vi "RT Main_Write Scalar.vi"() -> ()   [LabVIEW 2018]
uses:
  FPGA Bitfile Register Operations/Scalar IO Operations/TypeDefs/FXP Configuration.ctl
  <vilib>/fxp/LVFixedPointRepBitsTypeDef.ctl
  <vilib>/fxp/LVFixedPointRepRangeTypeDef.ctl
  FPGA Bitfile Register Operations/Scalar IO Operations/Write Methods/Write FXP.vi
  FPGA Bitfile Register Operations/Scalar IO Operations/Read Methods/Read FXP.vi
  <vilib>/FPGAPlugInAG/Dynamic/niLvFpga_Close_Dynamic.vi
  <vilib>/rvi/interface/nirviCloseFPGA/nirviCloseFPGA.xnode
  FPGA Bitfile Register Operations/Scalar IO Operations/Scalar IO Operations.lvlib
panel:
  in  "DBL Value Write":dbl=10.5 format="%#_13g"
  out "DBL Value Out":dbl
  out "Average seconds per write":dbl format="%#_6f"
  out "error out":errorcluster
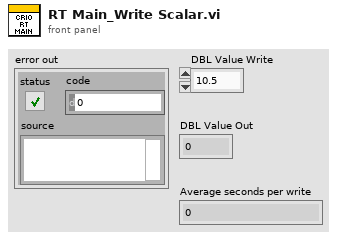
[diagram p1: front panel]
types:
  T1 = typedef "Scalar IO Operations.lvlib/FXP Configuration.ctl" = cluster{"FXP Representation":T2, "FXP Range":T3}
  T2 = typedef "LVFixedPointRepBitsTypeDef.ctl" = cluster{"Signed":bool, "Word Length":u32, "Integer Word Length":i32}
  T3 = typedef "LVFixedPointRepRangeTypeDef.ctl" = cluster{"Range Min":dbl, "Range Max":dbl, "Delta":dbl}
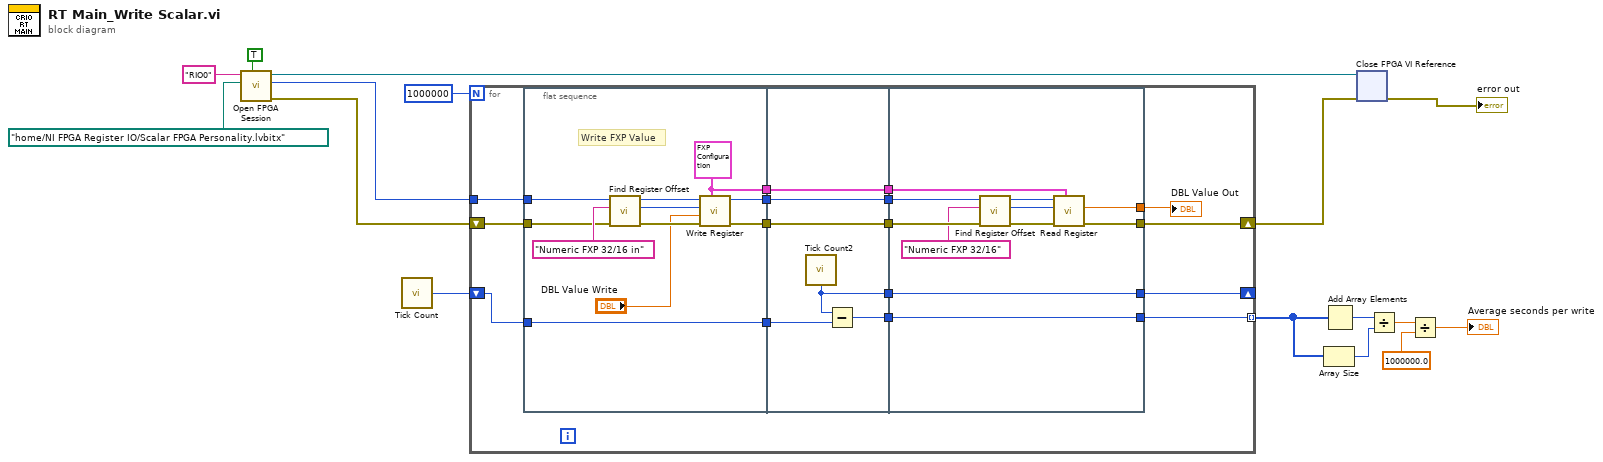
[diagram p0: block diagram]
diagram:
  n1 = call "Open FPGA Session.vi"("run when loaded (T)"=TRUE ("Run When Loaded (T)"), "bitfile path"=path "/home/NI FPGA Register IO/Scalar FPGA Personality.lvbitx" ("Bitfile path"), "device address"="RIO0" ("Device address")) -> ("error out"=w2:errorcluster, "session out"=w3:u64, "bitfile reference out"=w5:refnum<k20>)  [unwired: 6 in]
  n2 = call "Tick Count"() -> ("Tick Count(uSec)"=w12:u32)
  n3 = for {
    N: 1000000 -> [_]
    tunnel: w3 -> [w32]
    shift-right: [w30] -> w13
    shift-left: w2 -> [w31]
    shift-right: [w26] -> _
    shift-left: w12 -> [w28]
    tunnel: [w25] -> w11 mode=indexing
    n4 = flat-sequence {
      tunnel: w32 -> [w41]
      tunnel: w31 -> [w40]
      tunnel: [w39] -> w29
      tunnel: w28 -> [w43]
      tunnel: [w43] -> w27
      tunnel: [w34] -> w20
      tunnel: [w33] -> w19
      tunnel: w29 -> [w49]
      tunnel: w27 -> [w48]
      tunnel: [w49] -> w24
      tunnel: [w47] -> w23
      tunnel: [w46] -> w22
      tunnel: [w45] -> w21
      tunnel: w20 -> [w45]
      tunnel: w19 -> [w44]
      tunnel: [w44] -> w18
      tunnel: [w59] -> w25
      tunnel: [w60] -> w26
      tunnel: [w51] -> w30
      tunnel: w24 -> [w58]
      tunnel: w23 -> [w60]
      tunnel: w22 -> [w59]
      tunnel: w21 -> [w57]
      tunnel: w18 -> [w52]
      tunnel: [w50] -> w17
      frame #0 {
        w33 = T1 {"FXP Representation"={"Signed"=TRUE, "Word Length"=32, "Integer Word Length"=16}, "FXP Range"={"Range Min"=0.0, "Range Max"=0.0, "Delta"=1.52588e-05}} ("FXP Configuration")
        # "Write FXP Value"
        n5 = call "Find Register Offset.vi"("error in (no error)"=w40, "register name"="Numeric FXP 32/16 in" ("registerName"), "session in"=w41) -> ("error out"=w36:errorcluster, "resource offset"=w37:u32, "session out"=w38:u32)  [unwired: 6 in]
        n6 = call-poly "Write Register.vi"("FXP Configuration"=w33, "error in"=w36, "DBL Value"="DBL Value Write", "register offset"=w37, "session in"=w38) -> ("error out"=w39:errorcluster, "session out"=w34:u32)  [unwired: 5 in]
      }
      frame #1 {
        n7 = call "Tick Count2"() -> ("Tick Count(uSec)"=w47:u32)
        n8 = Subtract(x=w47, y=w48) -> (x-y=w46:u32)
      }
      frame #2 {
        n9 = call "Find Register Offset.vi"("error in (no error)"=w58, "register name"="Numeric FXP 32/16", "session in"=w57) -> ("error out"=w55:errorcluster, "resource offset"=w53:u32, "session out"=w54:u32)  [unwired: 6 in]
        n10 = call-poly "Read Register.vi"("FXP Configuration"=w52, "error in"=w55, "register offset"=w53, "session in"=w54) -> ("error out"=w51:errorcluster, "DBL Value"=w50:dbl)  [unwired: 5 in, 1 out]
      }
    }
    "DBL Value Out" <- w17
  }
  n11 = Array Size(array=w11) -> (size(s)=w9:i32)
  n12 = Add Array Elements(numeric array=w11) -> (sum=w10:u32)
  n13 = xnode "Close FPGA VI Reference"("FPGA VI Reference In"=w5, "error in"=w13) -> ("error out"=→"error out":errorcluster)
  n14 = Divide(x=w10, y=w9) -> (x/y=w8:dbl)
  n15 = Divide(x=w8, y=1000000.0) -> (x/y=→"Average seconds per write":dbl)
